vi "Keithley_close.vi"(7 "enable":bool, 8 "error in (no error)":errorcluster, 9 "Channel (Channel A) in":T1, 10 "Node Out":string, 11 "VISA Refnum in":refnum<visa-resource-name>) -> (0 "error out":errorcluster)   [LabVIEW 2012]
uses:
  Keithley 2600 Series/Keithley 2600 Series.lvlib
  Keithley 2600 Series/Public/Channel.ctl
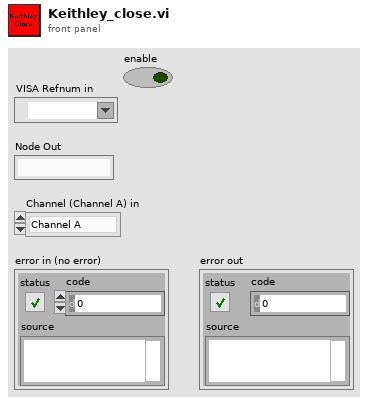
[diagram p1: front panel]
types:
  T1 = typedef "Keithley 2600 Series.lvlib/Channel.ctl" = enum32{"Channel A", "Channel B"}
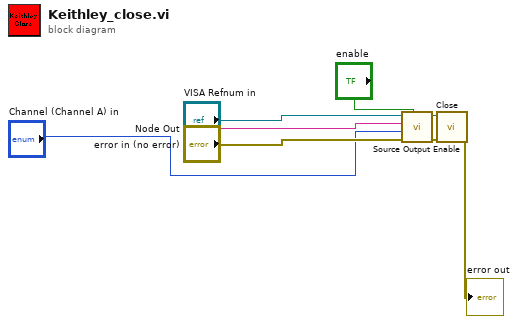
[diagram p0: block diagram]
diagram:
  n1 = call "Source Output Enable.vi"("Output (Off)"="enable", "error in (no error)"="error in (no error)", "Channel (Channel A)"="Channel (Channel A) in", "Node In"="Node Out", "VISA resource name"="VISA Refnum in") -> ("error out"=w1:errorcluster, "VISA resource name out"=w2:refnum<visa-resource-name>)  [unwired: 5 out]
  n2 = call "Close.vi"("error in (no error)"=w1, "VISA resource name"=w2) -> ("error out"=→"error out":errorcluster)  [unwired: 9 out]
